vi "Read AccountNumber.vi"(8 "error in (no error)":errorcluster, 11 "AWS_SQS in":refnum<class "AWS_SQS.lvclass">) -> (0 "error out":errorcluster, 2 "AccountNumber":string, 3 "AWS_SQS out":refnum<class "AWS_SQS.lvclass">)   [LabVIEW 2015, in "AWS_SQS.lvlib" / "AWS_SQS.lvclass"]
uses:
  AWS_SQS.lvclass
  AWS_SQS.lvclass/AWS_SQS.ctl
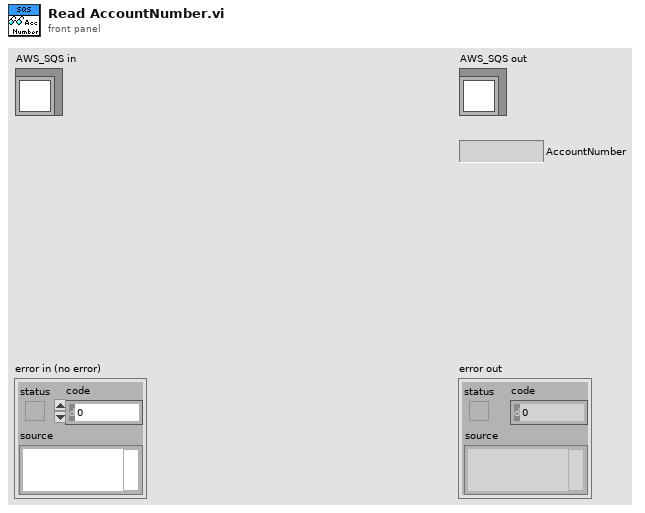
[diagram p1: front panel]
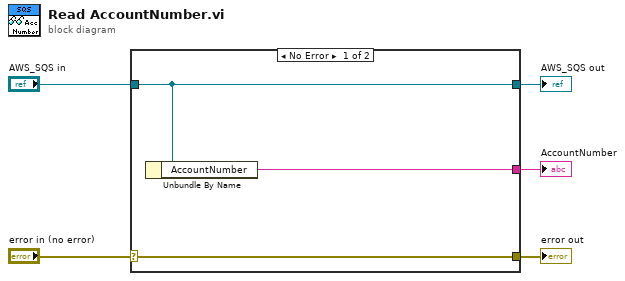
[diagram p0: block diagram]
diagram:
  n1 = case shown="No Error" "error in (no error)" {
    selector: "error in (no error)" -> [w8 w9]
    tunnel: [w8 w9] -> w4
    tunnel: [w7 w10] -> w2
    tunnel: "AWS_SQS in" -> [w7 w10]
    tunnel: [w6 _] -> w1
    frame No Error {
      n2 = Unbundle By Name(w7) -> ("AccountNumber"=w6:string)
    }
    frame Error {
    }
  }
  "error out" <- w4
  "AWS_SQS out" <- w2
  "AccountNumber" <- w1
